vi "Gergberg v4.vi"() -> ()   [LabVIEW 2012, in "LightPipes.lvlib"]
uses:
  LightPipes.lvlib
panel:
  in  "Forward Distance":dbl(slide) step=0.0001 scale=-0.02..0.02
  in  "stop":bool
  out "Distance":dbl
  out "Iteration":i32
  out "Original Far Field":T1(plugin-control)
  out "Original Mid Field":T1(plugin-control)
  out "error out":errorcluster
  in  "error in (no error)":errorcluster
  in  "field":T2
  out "Far Field":T1(plugin-control)
  out "MF Phase":T1(plugin-control)
  out "Target Intensity\n RMS Error":dbl(graph)=4.212939404164251
  out "FF Phase":T1(plugin-control)
  out "Mid Field":T1(plugin-control)
  in  "n_grid":i32=300
  in  "lambda":dbl=1.054e-06
  in  "forward distance":dbl=0.02
  in  "size_grid":dbl=0.001776
  in  "Number of Iteration":i32=10
  in  "Far Field":path=path "C:/Users/Tri/Documents/Lightpipes/LabView/beam images/Centered FF.png"
  in  "Mid Field":path=path "C:/Users/Tri/Documents/Lightpipes/LabView/beam images/Centered MF.png"
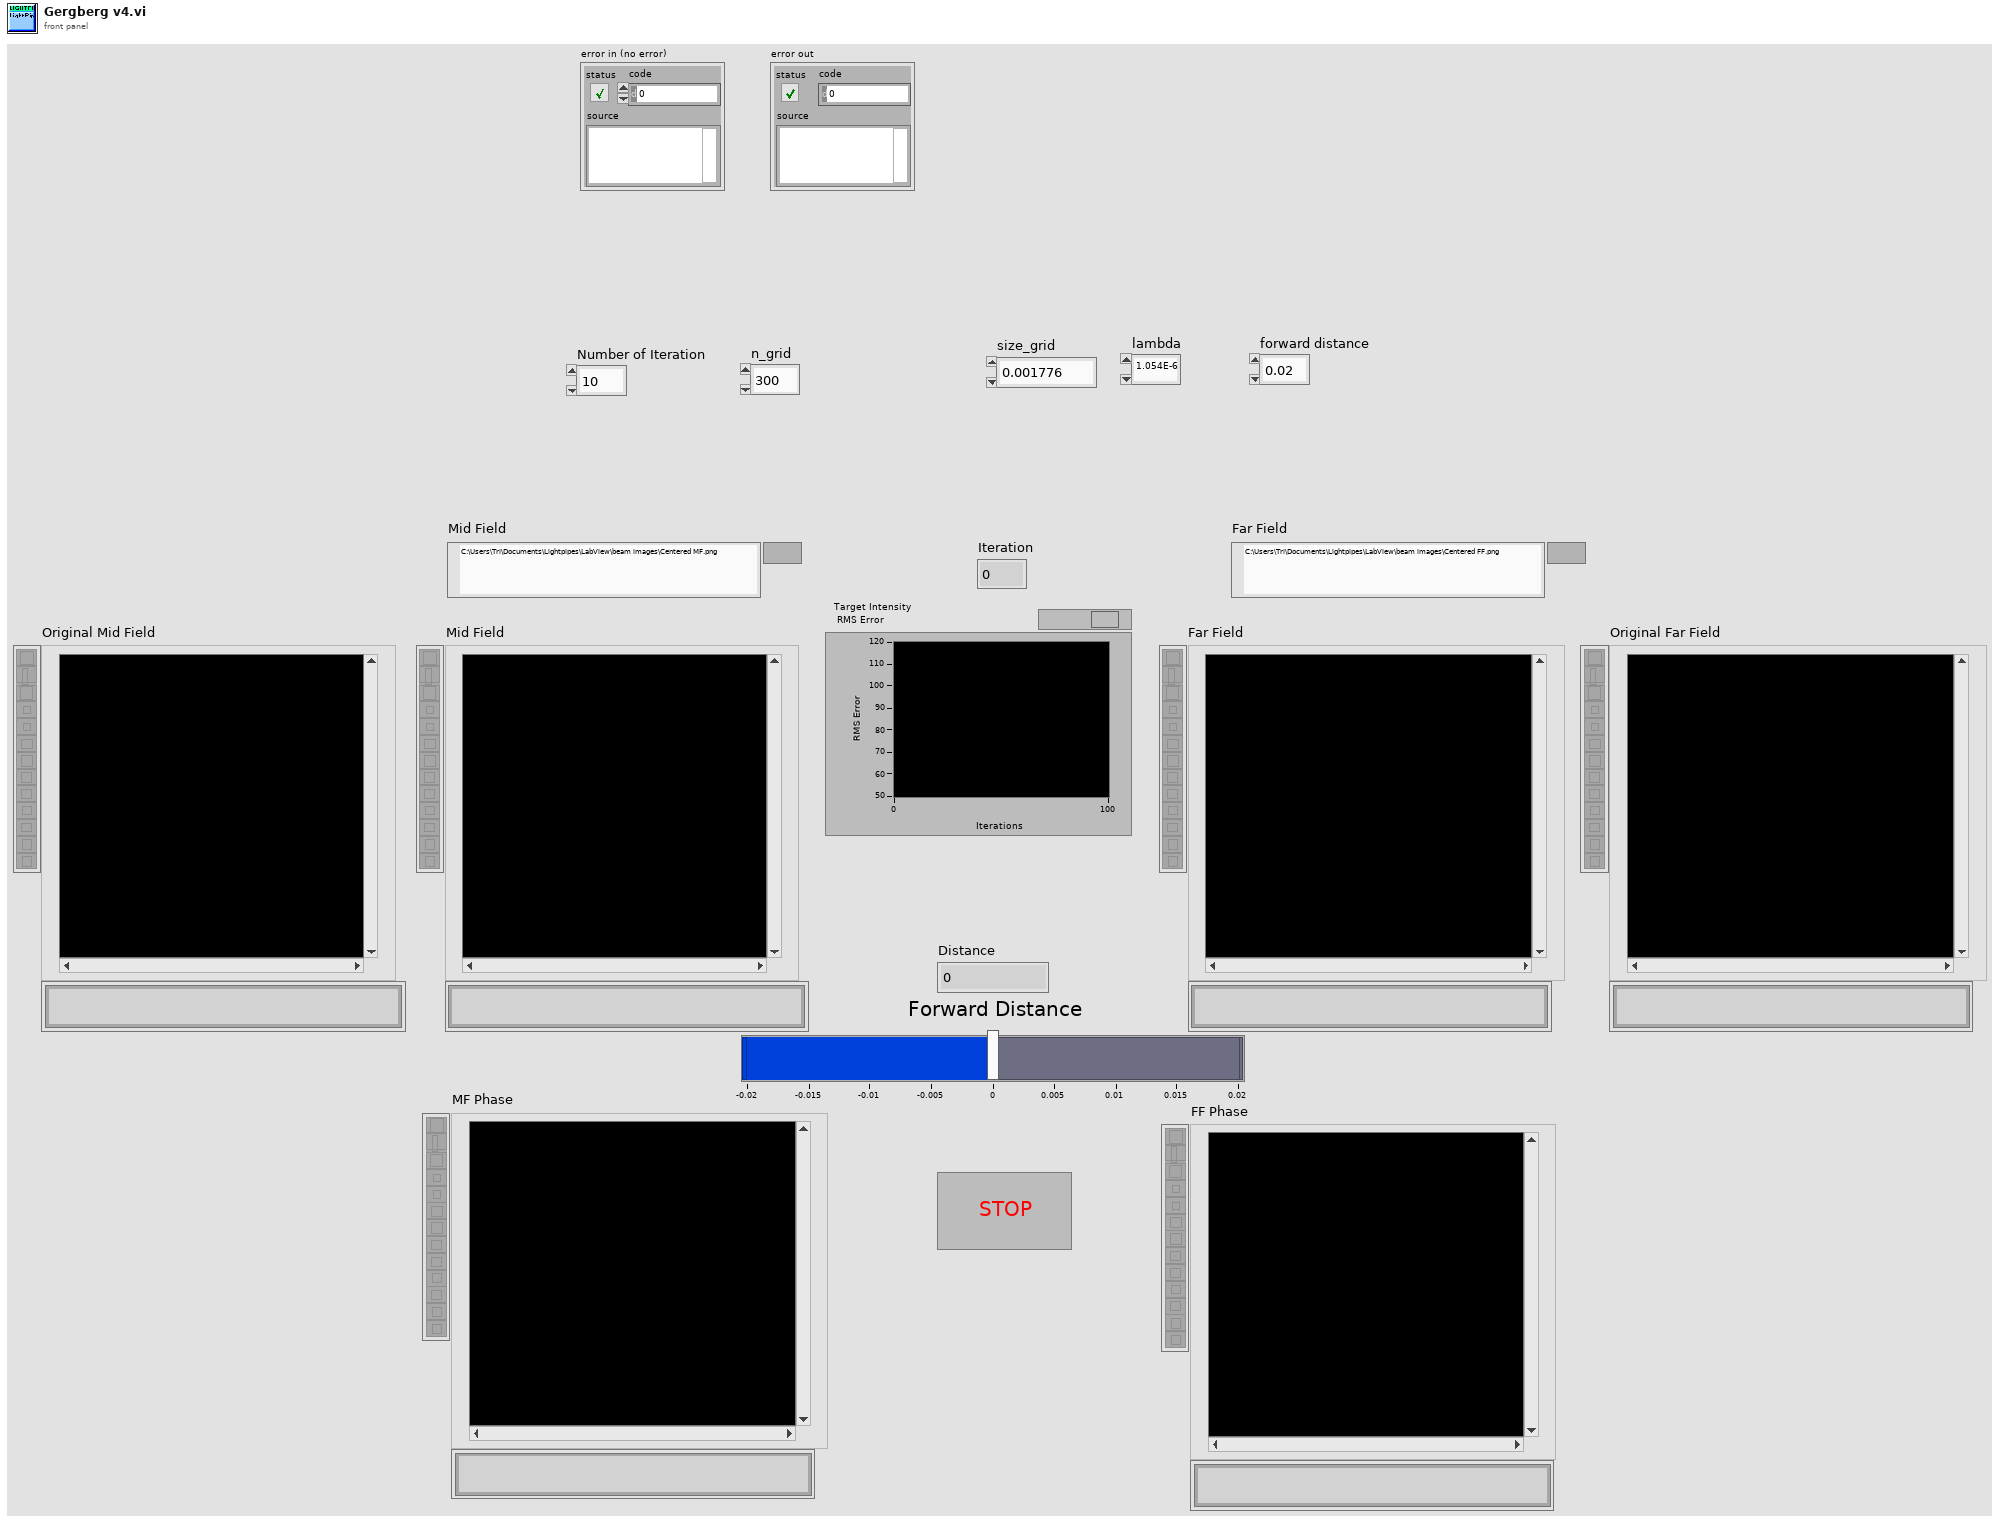
[diagram p1: front panel]
types:
  T1 = typedef "IMAQ Image.ctl" = refnum<image>
  T2 = cluster{"n_grid":i32, "@dummy control@":i8, "@dummy control@":i8, "@dummy control@":i8, "@dummy control@":i8, "size":dbl, "lambda":dbl, "int1":i32, "int2":i32, "int3":i32, "@dummy control@":i8, "@dummy control@":i8, "@dummy control@":i8, "@dummy control@":i8, "double1":dbl, "double2":dbl, "double3":dbl, "real":u32, "imaginary":u32}
  T3 = typedef "Image Type" = u32
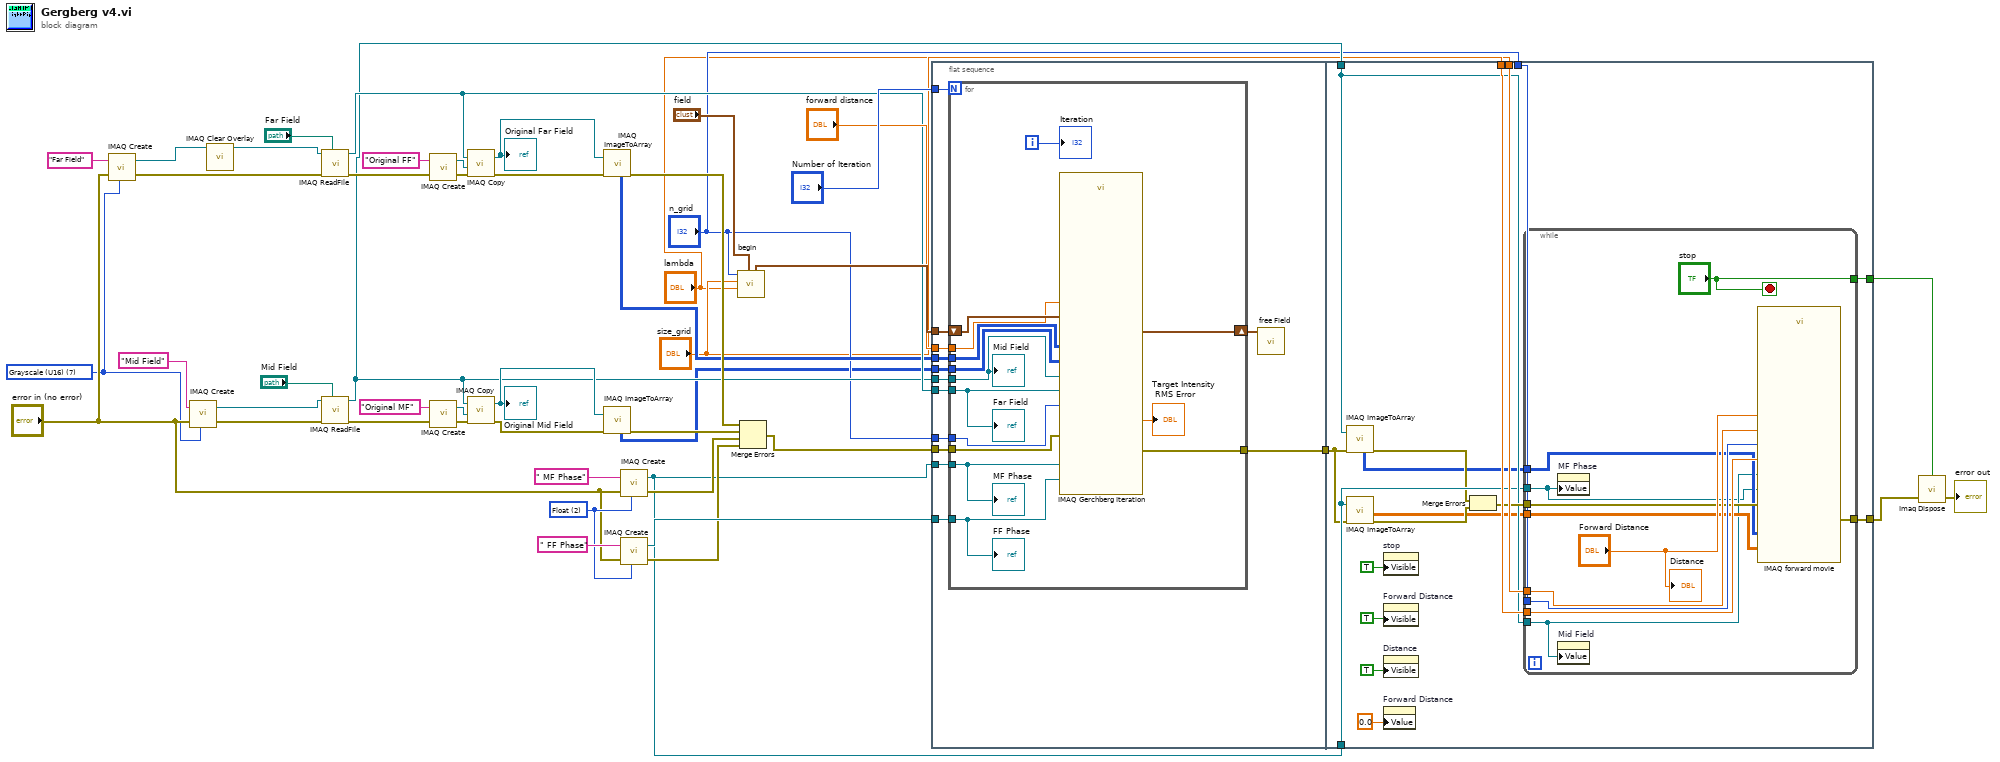
[diagram p0: block diagram]
diagram:
  w11 = T3 7 items=["Grayscale (U8)", "Grayscale (I16)", "Grayscale (SGL)", "Complex (CSG)", "RGB (U32)", "HSL (U32)", "RGB (U64)", "Grayscale (U16)"] ("Image Type")
  w41 = u32 2 items=["8 bits", "16 bits", "Float", "Complex", "RGB", "HSL"] ("Image Type")
  n1 = call "IMAQ Create"("Image Name"="Far Field", "Image Type"=w11, "error in (no error)"="error in (no error)") -> ("New Image"=w15:T1, "error out"=w27:errorcluster)  [unwired: 2 in]
  n2 = call "IMAQ Create"("Image Name"="Mid Field", "Image Type"=w11, "error in (no error)"="error in (no error)") -> ("New Image"=w42:T1, "error out"=w25:errorcluster)  [unwired: 2 in]
  n3 = call "IMAQ Clear Overlay"("Image"=w15) -> ("Image Out"=w14:T1)  [unwired: 9 in, 1 out]
  n4 = call "IMAQ ReadFile"("File Path"="Far Field", "error in (no error)"=w27, "Image"=w14) -> ("error out"=w26:errorcluster, "Image Out"=w28:T1)  [unwired: 2 in, 5 out]
  n5 = call "IMAQ ReadFile"("File Path"="Mid Field", "error in (no error)"=w25, "Image"=w42) -> ("error out"=w24:errorcluster, "Image Out"=w6:T1)  [unwired: 2 in, 5 out]
  n6 = call "IMAQ Create"("Image Name"="Original FF", "error in (no error)"=w26) -> ("New Image"=w37:T1, "error out"=w36:errorcluster)  [unwired: 3 in]
  n7 = call "IMAQ Create"("Image Name"="Original MF", "error in (no error)"=w24) -> ("New Image"=w40:T1, "error out"=w39:errorcluster)  [unwired: 3 in]
  n8 = call "IMAQ Copy"("error in (no error)"=w36, "Image Dst"=w37, "Image Src"=w28) -> ("error out"=w30:errorcluster, "Image Dst Out"=w16:T1)  [unwired: 3 in]
  "Original Far Field" <- w16
  n9 = call "IMAQ Copy"("error in (no error)"=w39, "Image Dst"=w40, "Image Src"=w6) -> ("error out"=w29:errorcluster, "Image Dst Out"=w17:T1)  [unwired: 3 in]
  "Original Mid Field" <- w17
  n10 = call "IMAQ ImageToArray"("error in (no error)"=w30, "Image"=w16) -> ("Image Pixels (U16)"=w12:u16[][], "error out"=w23:errorcluster)  [unwired: 2 in, 3 out]
  n11 = call "IMAQ ImageToArray"("error in (no error)"=w29, "Image"=w17) -> ("Image Pixels (U16)"=w1:u16[][], "error out"=w22:errorcluster)  [unwired: 2 in, 3 out]
  n12 = call "IMAQ Create"("Image Name"=" MF Phase", "Image Type"=w41, "error in (no error)"="error in (no error)") -> ("New Image"=w7:T1, "error out"=w19:errorcluster)  [unwired: 2 in]
  n13 = call "IMAQ Create"("Image Name"=" FF Phase", "Image Type"=w41, "error in (no error)"="error in (no error)") -> ("New Image"=w20:T1, "error out"=w18:errorcluster)  [unwired: 2 in]
  n14 = call "begin.vi"("field"="field", "lambda"="lambda", "size_grid"="size_grid", "n_grid"="n_grid") -> ("field out"=w32:T2)  [unwired: 7 in]
  n15 = Merge Errors(w23, w22, w19, w18) -> (w21:errorcluster)
  n16 = flat-sequence {
    tunnel: "Number of Iteration" -> [w61]
    tunnel: w32 -> [w60]
    tunnel: "forward distance" -> [w59]
    tunnel: w6 -> [w57]
    tunnel: w28 -> [w56]
    tunnel: w21 -> [w55]
    tunnel: "n_grid" -> [w54]
    tunnel: w20 -> [w53]
    tunnel: w7 -> [w52]
    tunnel: w1 -> [w51]
    tunnel: w12 -> [w50]
    tunnel: [w49] -> w10
    tunnel: w10 -> [w80]
    tunnel: [w90] -> w8
    tunnel: w7 -> [w81]
    tunnel: w6 -> [w82]
    tunnel: "n_grid" -> [w89]
    tunnel: "size_grid" -> [w88]
    tunnel: "lambda" -> [w87]
    tunnel: [w86] -> w2
    frame #0 {
      n17 = for {
        N: w61 -> [_]
        shift-right: [w74] -> w58
        shift-left: w60 -> [w75]
        tunnel: w59 -> [w73]
        tunnel: w51 -> [w68]
        tunnel: w50 -> [w69]
        tunnel: w57 -> [w66]
        tunnel: w56 -> [w65]
        tunnel: w55 -> [w72]
        tunnel: [w71] -> w49
        tunnel: w54 -> [w70]
        tunnel: w53 -> [w62]
        tunnel: w52 -> [w63]
        i -> [w67]
        n18 = call "IMAQ Gerchberg Iteration.vi"("field"=w75, "Original Source (U16)"=w68, "n_grid"=w70, "forward distance"=w73, "Original Target (U16)"=w69, "error in (no error)"=w72, "Source"=w66, "Target"=w65, "Source Phase"=w63, "Target Phase"=w62) -> ("field out"=w74:T2, "Target Intensity\n RMS Error"=→"Target Intensity\n RMS Error":dbl, "error out"=w71:errorcluster)  [unwired: 7 in]
        "Iteration" <- w67
        "Mid Field" <- w66
        "Far Field" <- w65
        "MF Phase" <- w63
        "FF Phase" <- w62
      }
      n19 = call "free Field.vi"("field"=w58) -> ()  [unwired: 10 in, 1 out]
    }
    frame #1 {
      n20 = call "IMAQ ImageToArray"("error in (no error)"=w80, "Image"=w82) -> ("Image Pixels (U16)"=w76:u16[][], "error out"=w79:errorcluster)  [unwired: 2 in, 3 out]
      n21 = call "IMAQ ImageToArray"("error in (no error)"=w80, "Image"=w81) -> ("Image Pixels (Float)"=w77:sgl[][], "error out"=w78:errorcluster)  [unwired: 2 in, 3 out]
      n22 = property on="stop" class="Bool"("Visible"=TRUE) -> ()  [unwired: 2 in, 2 out]
      n23 = property on="Forward Distance" class="Slide (strict)"("Visible"=TRUE) -> ()  [unwired: 2 in, 2 out]
      n24 = property on="Distance" class="DigNum (strict)"("Visible"=TRUE) -> ()  [unwired: 2 in, 2 out]
      n25 = property on="Forward Distance" class="Slide (strict)"("Value"=0.0 ("Forward Distance")) -> ()  [unwired: 2 in, 2 out]
      n26 = Merge Errors(w79, w78) -> (w85:errorcluster)
      n27 = while {
        tunnel: ["stop"] -> w90
        tunnel: w81 -> [w93]
        tunnel: w82 -> [w94]
        tunnel: w89 -> [w102]
        tunnel: w88 -> [w101]
        tunnel: w87 -> [w100]
        tunnel: [w97] -> w86
        tunnel: w85 -> [w98]
        tunnel: w76 -> [w96]
        tunnel: w77 -> [w95]
        stop <- "stop" stop-if-true
        n28 = property on="MF Phase" class="ImageControl"("Value"=w93) -> ()  [unwired: 2 in, 2 out]
        n29 = property on="Mid Field" class="ImageControl"("Value"=w94) -> ()  [unwired: 2 in, 2 out]
        n30 = call "IMAQ forward movie.vi"("Forwarded Phase"=w93, "n_grid"=w102, "Source Intensity (U16)"=w96, "Forwarded Intensity"=w94, "error in (no error)"=w98, "size_grid"=w101, "lambda"=w100, "Forward Distance"="Forward Distance", "Source Phase (Float)"=w95) -> ("error out"=w97:errorcluster)  [unwired: 6 in]
        "Distance" <- "Forward Distance"
      }
    }
  }
  n31 = call "Imaq Dispose"("All Images? (No)"=w8, "error in (no error)"=w2) -> ("error out"=→"error out":errorcluster)  [unwired: 4 in]
